vi "Get Value by pointer.vi"() -> ()   [LabVIEW 2012]
uses:
  <vilib>/Utility/importsl/GetValueByPointer/datatype.ctl
  <vilib>/Utility/importsl/GetValueByPointer/GetValueByPointer.xnode
  demo dll.dll
panel:
  out "Output":cluster{"U8":u8, "I32":i32, "DBL":dbl}
  in  "Pack1Cluster":cluster{"U8":u8, "I32":i32, "DBL":dbl}
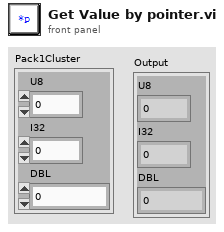
[diagram p1: front panel]
types:
  T1 = enum32{"pack1", "pack2", "pack4", "pack8", "pack16"}
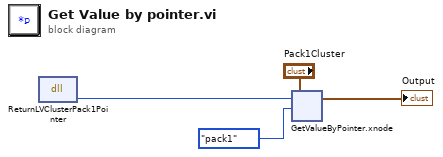
[diagram p0: block diagram]
diagram:
  n1 = dll-call lib="PTH1+abs EBOOK\t功能块DLLdemo dll.dll" fn="ReturnLVClusterPack1Pointer"() -> ("返回类型"=w4:u64)  [unwired: 3 in, 2 out]
  n2 = xnode "GetValueByPointer.xnode"("Pointer"=w4, "InputType"="Pack1Cluster", "PackType"=T1."pack1") -> ("Output"=→"Output":cluster{"U8":u8, "I32":i32, "DBL":dbl})  [unwired: 1 in, 1 out]
